vi "Main.vi"   [LabVIEW 2020, in "HAL Config.lvlib" / "HAL Editor.lvclass"]
uses:
  HAL Editor.lvclass
panel:
  # "Config\nEditor\nMain"
types:
  T1 = enum32{"Invalid", "Standard", "Closed", "Hidden", "Minimized", "Maximized"}
  T2 = enum32{"invalid app kind", "Development System", "Run Time System", "Student Edition", "Embedded LabVIEW", "Evaluation", "Custom", "Community Edition"}
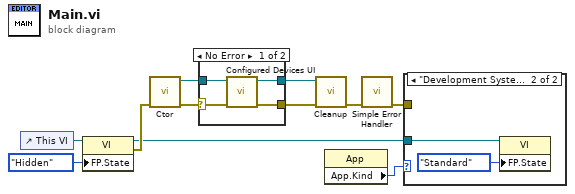
[diagram p0: block diagram]
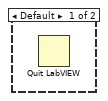
[diagram p3: hidden frame]
diagram:
  n1 = control-ref of="This VI"() -> (w11:refnum<vi>)
  n2 = property class="VI"(reference=w11, "FP.State"=T1."Hidden" ("Front Panel Window:State")) -> (reference out=w1:refnum<vi>, error out=w9:errorcluster)  [unwired: 1 in]
  n3 = call "Ctor.vi"("error in (no error)"=w9) -> ("error out"=w8:errorcluster, "HAL Editor out"=w7:refnum<class "HAL Editor.lvclass">)  [unwired: 9 in]
  n4 = case shown="No Error" w8 {
    selector: w8 -> [w15 w17]
    tunnel: w7 -> [w14 w16]
    tunnel: [w13 w17] -> w6
    tunnel: [w12 w16] -> w5
    frame No Error {
      n5 = call "Configured Devices UI.vi"("error in (no error)"=w15, "HAL Editor in"=w14) -> ("error out"=w13:errorcluster, "HAL Editor out"=w12:refnum<class "HAL Editor.lvclass">)  [unwired: 8 in]
    }
    frame Error {
    }
  }
  n6 = call "Cleanup.vi"("error in (no error)"=w6, "HAL Editor in"=w5) -> ("error out"=w4:errorcluster)  [unwired: 9 in]
  n7 = property class="App"() -> ("App.Kind"=w2:T2)  [unwired: 2 in, 2 out]
  n8 = call <vilib>:"Simple Error Handler.vi"("error in (no error)"=w4) -> ("error out"=w3:errorcluster)  [unwired: 4 in, 4 out]
  n9 = case shown="\"Development System\"" w2 {
    tunnel: w3 -> [_ _]
    tunnel: w1 -> [_ w18]
    frame Default {
      n10 = Quit LabVIEW() -> ()  [unwired: 1 in]
    }
    frame "Development System" {
      n11 = property class="VI"(reference=w18, "FP.State"=T1."Standard" ("Front Panel Window:State")) -> ()  [unwired: 1 in, 2 out]
    }
  }
